vi "Image_UART.vi"() -> ()   [LabVIEW 2018]
uses:
  <vilib>/myRIO/Instrument Drivers/Onboard IO/UART/typedef/VISA Configuration.ctl
  <vilib>/Instr/_visa.llb/VISA Configure Serial Port (Instr).vi
  <vilib>/picture/picture.llb/Draw True-Color Pixmap.vi
  <vilib>/myRIO/Express VI/Onboard IO/UART/UART Express VI.xnode
  <vilib>/myRIO/Instrument Drivers/Onboard IO/UART/UART.lvlib
panel:
  out "new picture":picture
  in  "stop":bool
  out "s? t:f":string[](array[string])
  out "Characters Read":string
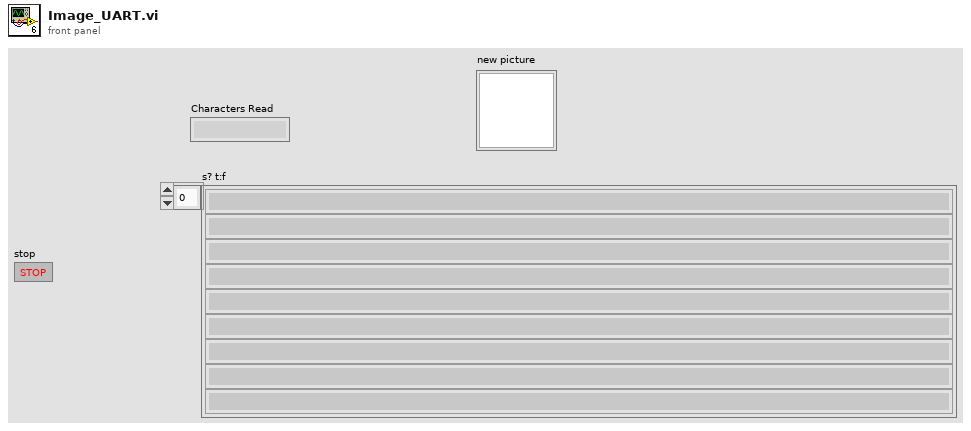
[diagram p1: front panel]
types:
  T1 = typedef "UART.lvlib/VISA Configuration.ctl" = cluster{"baud rate (9600)":u32, "data bits (8)":u16, "parity (0:none)":enum16{"None", "Odd", "Even", "Mark", "Space"}, "stop bits (10: 1 bit)":u16, "flow control (0:none)":u16, "termination char\n(0xA = '\\n' = LF) ":u8, "Enable Termination\nChar (T)":bool, "timeout (10sec)":u32}
  T2 = typedef "IMAQ Image.ctl" = refnum<image>
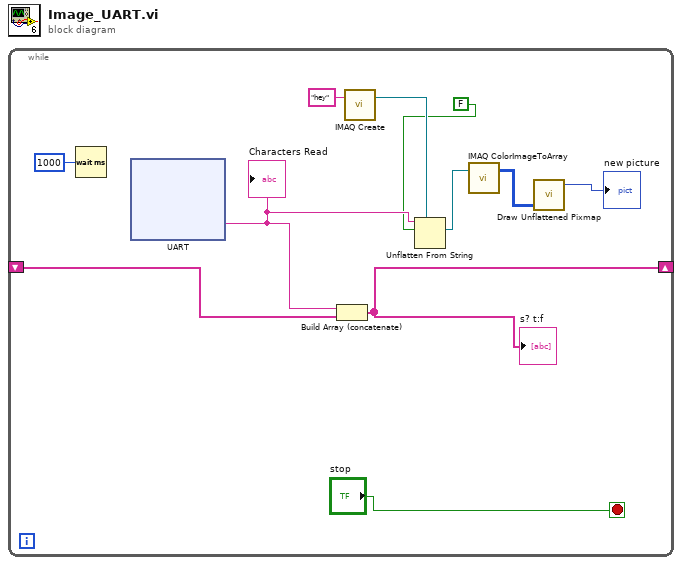
[diagram p0: block diagram]
diagram:
  n1 = while {
    shift-right: [w8] -> _
    shift-left: _ -> [w9]
    stop <- "stop" stop-if-true
    n2 = Wait (ms)(milliseconds to wait=u32 1000) -> ()  [unwired: 1 out]
    n3 = xnode "UART"() -> ("Characters Read"=w7:string)  [unwired: 1 in, 1 out]
    "Characters Read" <- w7
    n4 = Build Array (concatenate)(w7, w9) -> (w8:string[])
    "s? t:f" <- w8
    n5 = call "IMAQ Create"("Image Name"="hey") -> ("New Image"=w4:T2)  [unwired: 4 in, 1 out]
    n6 = Unflatten From String(type=w4, binary string=w7, data includes array or string size? (T)=FALSE) -> (value=w2:T2)  [unwired: 2 in, 2 out]
    n7 = call "IMAQ ColorImageToArray"("Image"=w2) -> ("Image Pixels (U32)"=w6:u32[][])  [unwired: 3 in, 2 out]
    n8 = call-poly <vilib>:"Draw Unflattened Pixmap.vi"("data (RGB format)"=w6) -> ("new picture"=→"new picture":picture)  [unwired: 8 in]
  }
